vi "ScanDelaySetScannerOffset.vi"(8 "error in (no error)":errorcluster, 9 "wait":u32=10, 10 "value":dbl, 11 "VISA resource name in":refnum<visa-resource-name>) -> (0 "error out":errorcluster, 3 "VISA resource name out":refnum<visa-resource-name>)   [LabVIEW 2018]
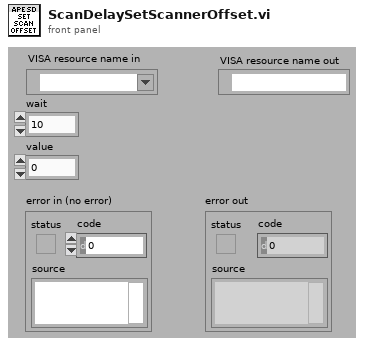
[diagram p1: front panel]
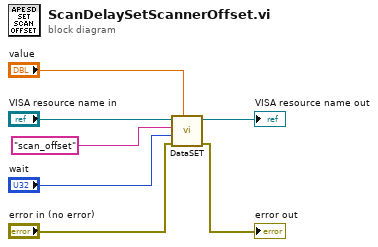
[diagram p0: block diagram]
diagram:
  n1 = call "DataSET.vi"("value"="value", "error in"="error in (no error)", "wait"="wait", "parameter"="scan_offset", "VISA resource name"="VISA resource name in") -> ("error out"=→"error out":errorcluster, "VISA resource name out"=→"VISA resource name out":refnum<visa-resource-name>)  [unwired: 5 in]
